vi "Weather Parse Test.vi"() -> ()   [LabVIEW 2020, in "CDM-Config.lvlib"] (continued)
        },\n                \"affectedZones\": [\n                    \"https://api.weather.gov/zones/forecast/PKZ760\"\n                ],\n                \"references\": [],\n                \"sent\": \"2025-12-03T04:00:00-09:00\",\n                \"effective\": \"2025-12-03T04:00:00-09:00\",\n                \"onset\": \"2025-12-03T04:00:00-09:00\",\n                \"expires\": \"2025-12-03T17:00:00-09:00\",\n                \"ends\": \"2025-12-04T17:00:00-09:00\",\n                \"status\": \"Actual\",\n                \"messageType\": \"Alert\",\n                \"category\": \"Met\",\n                \"severity\": \"Minor\",\n                \"certainty\": \"Likely\",\n                \"urgency\": \"Expected\",\n                \"event\": \"Small Craft Advisory\",\n                \"sender\": \"w-nws.webmaster@noaa.gov\",\n                \"senderName\": \"NWS Anchorage AK\",\n                \"headline\": \"Small Craft Advisory issued December 3 at 4:00AM AKST until December 4 at 5:00PM AKST by NWS Anchorage AK\",\n                \"description\": \"Coastal Waters Forecast for Southwest Alaska+Bristol Bay+The\\nAlaska Peninsula Waters and the Aleutian Islands up to 100 nm out.\\n\\nWind forecasts reflect the predominant speed and direction\\nexpected. Sea forecasts represent an average of the highest\\none-third of the combined wind wave and swell height.\\n\\n.TODAY...E wind 25 kt. Seas 5 ft.\\n.TONIGHT...E wind 30 kt. Seas 5 ft. Rain showers.\\n.THU...NE wind 30 kt. Seas 7 ft.\\n.THU NIGHT...NE wind 25 kt. Seas 7 ft.\\n.FRI...N wind 30 kt. Seas 6 ft.\\n.SAT...N wind 35 kt. Seas 9 ft.\\n.SUN...N wind 30 kt. Seas 7 ft.\",\n                \"instruction\": null,\n                \"response\": \"Avoid\",\n                \"parameters\": {\n                    \"AWIPSidentifier\": [\n                        \"CWFALU\"\n                    ],\n                    \"WMOidentifier\": [\n                        \"FZAK52 PAFC 031300\"\n                    ],\n                    \"NWSheadline\": [\n                        \"SMALL CRAFT ADVISORY THROUGH THURSDAY\"\n                    ],\n                    \"BLOCKCHANNEL\": [\n                        \"EAS\",\n                        \"NWEM\",\n                        \"CMAS\"\n                    ],\n                    \"VTEC\": [\n                        \"/O.NEW.PAFC.SC.Y.5665.251203T1300Z-251205T0200Z/\"\n                    ],\n                    \"eventEndingTime\": [\n                        \"2025-12-04T17:00:00-09:00\"\n                    ]\n                },\n                \"scope\": \"Public\",\n                \"code\": \"IPAWSv1.0\",\n                \"language\": \"en-US\",\n                \"web\": \"http://www.weather.gov\",\n                \"eventCode\": {\n                    \"SAME\": [\n                        \"NWS\"\n                    ],\n                    \"NationalWeatherService\": [\n                        \"SCY\"\n                    ]\n                }\n            }\n        },\n        {\n            \"id\": \"https://api.weather.gov/alerts/urn:oid:2.49.0.1.840.0.16ee1729296b80b5948b72c512c8722f6075ae6c.032.1\",\n            \"type\": \"Feature\",\n            \"geometry\": null,\n            \"properties\": {\n                \"@id\": \"https://api.weather.gov/alerts/urn:oid:2.49.0.1.840.0.16ee1729296b80b5948b72c512c8722f6075ae6c.032.1\",\n                \"@type\": \"wx:Alert\",\n                \"id\": \"urn:oid:2.49.0.1.840.0.16ee1729296b80b5948b72c512c8722f6075ae6c.032.1\",\n                \"areaDesc\": \"Bristol Bay from Cape Chichagof to Cape Pierce out to 15 NM\",\n                \"geocode\": {\n                    \"SAME\": [\n                        \"058762\"\n                    ],\n                    \"UGC\": [\n                        \"PKZ762\"\n                    ]\n                },\n                \"affectedZones\": [\n                    \"https://api.weather.gov/zones/forecast/PKZ762\"\n                ],\n                \"references\": [],\n                \"sent\": \"2025-12-03T04:00:00-09:00\",\n                \"effective\": \"2025-12-03T04:00:00-09:00\",\n                \"onset\": \"2025-12-03T17:00:00-09:00\",\n                \"expires\": \"2025-12-03T17:00:00-09:00\",\n                \"ends\": \"2025-12-04T17:00:00-09:00\",\n                \"status\": \"Actual\",\n                \"messageType\": \"Alert\",\n                \"category\": \"Met\",\n                \"severity\": \"Minor\",\n                \"certainty\": \"Likely\",\n                \"urgency\": \"Expected\",\n                \"event\": \"Small Craft Advisory\",\n                \"sender\": \"w-nws.webmaster@noaa.gov\",\n                \"senderName\": \"NWS Anchorage AK\",\n                \"headline\": \"Small Craft Advisory issued December 3 at 4:00AM AKST until December 4 at 5:00PM AKST by NWS Anchorage AK\",\n                \"description\": \"Coastal Waters Forecast for Southwest Alaska+Bristol Bay+The\\nAlaska Peninsula Waters and the Aleutian Islands up to 100 nm out.\\n\\nWind forecasts reflect the predominant speed and direction\\nexpected. Sea forecasts represent an average of the highest\\none-third of the combined wind wave and swell height.\\n\\n.TODAY...NE wind 20 kt. Seas 3 ft.\\n.TONIGHT...NE wind 25 kt. Seas 4 ft. Rain showers.\\n.THU...NE wind 25 kt. Seas 4 ft.\\n.THU NIGHT...NE wind 25 kt. Seas 4 ft.\\n.FRI...N wind 30 kt. Seas 4 ft.\\n.SAT...N wind 35 kt. Seas 5 ft.\\n.SUN...N wind 30 kt. Seas 3 ft.\",\n                \"instruction\": null,\n                \"response\": \"Avoid\",\n                \"parameters\": {\n                    \"AWIPSidentifier\": [\n                        \"CWFALU\"\n                    ],\n                    \"WMOidentifier\": [\n                        \"FZAK52 PAFC 031300\"\n                    ],\n                    \"NWSheadline\": [\n                        \"SMALL CRAFT ADVISORY TONIGHT AND THURSDAY\"\n                    ],\n                    \"BLOCKCHANNEL\": [\n                        \"EAS\",\n                        \"NWEM\",\n                        \"CMAS\"\n                    ],\n                    \"VTEC\": [\n                        \"/O.NEW.PAFC.SC.Y.5666.251204T0200Z-251205T0200Z/\"\n                    ],\n                    \"eventEndingTime\": [\n                        \"2025-12-04T17:00:00-09:00\"\n                    ]\n                },\n                \"scope\": \"Public\",\n                \"code\": \"IPAWSv1.0\",\n                \"language\": \"en-US\",\n                \"web\": \"http://www.weather.gov\",\n                \"eventCode\": {\n                    \"SAME\": [\n                        \"NWS\"\n                    ],\n                    \"NationalWeatherService\": [\n                        \"SCY\"\n                    ]\n                }\n            }\n        },\n        {\n            \"id\": \"https://api.weather.gov/alerts/urn:oid:2.49.0.1.840.0.16ee1729296b80b5948b72c512c8722f6075ae6c.011.1\",\n            \"type\": \"Feature\",\n            \"geometry\": null,\n            \"properties\": {\n                \"@id\": \"https://api.weather.gov/alerts/urn:oid:2.49.0.1.840.0.16ee1729296b80b5948b72c512c8722f6075ae6c.011.1\",\n                \"@type\": \"wx:Alert\",\n                \"id\": \"urn:oid:2.49.0.1.840.0.16ee1729296b80b5948b72c512c8722f6075ae6c.011.1\",\n                \"areaDesc\": \"Nelson Lagoon to Cape Sarichef from 15 to 70 NM\",\n                \"geocode\": {\n                    \"SAME\": [\n                        \"058759\"\n                    ],\n                    \"UGC\": [\n                        \"PKZ759\"\n                    ]\n                },\n                \"affectedZones\": [\n                    \"https://api.weather.gov/zones/forecast/PKZ759\"\n                ],\n                \"references\": [],\n                \"sent\": \"2025-12-03T04:00:00-09:00\",\n                \"effective\": \"2025-12-03T04:00:00-09:00\",\n                \"onset\": \"2025-12-03T04:00:00-09:00\",\n                \"expires\": \"2025-12-03T17:00:00-09:00\",\n                \"ends\": \"2025-12-04T17:00:00-09:00\",\n                \"status\": \"Actual\",\n                \"messageType\": \"Alert\",\n                \"category\": \"Met\",\n                \"severity\": \"Minor\",\n                \"certainty\": \"Likely\",\n                \"urgency\": \"Expected\",\n                \"event\": \"Small Craft Advisory\",\n                \"sender\": \"w-nws.webmaster@noaa.gov\",\n                \"senderName\": \"NWS Anchorage AK\",\n                \"headline\": \"Small Craft Advisory issued December 3 at 4:00AM AKST until December 4 at 5:00PM AKST by NWS Anchorage AK\",\n                \"description\": \"Coastal Waters Forecast for Southwest Alaska+Bristol Bay+The\\nAlaska Peninsula Waters and the Aleutian Islands up to 100 nm out.\\n\\nWind forecasts reflect the predominant speed and direction\\nexpected. Sea forecasts represent an average of the highest\\none-third of the combined wind wave and swell height.\\n\\n.TODAY...E wind 25 kt. Seas 9 ft. Rain showers.\\n.TONIGHT...NE wind 30 kt. Seas 11 ft. Rain showers.\\n.THU...NE wind 25 kt. Seas 12 ft.\\n.THU NIGHT...NE wind 25 kt. Seas 9 ft.\\n.FRI...NE wind 35 kt. Seas 12 ft.\\n.SAT...N wind 40 kt. Seas 17 ft.\\n.SUN...N wind 35 kt. Seas 16 ft.\",\n                \"instruction\": null,\n                \"response\": \"Avoid\",\n                \"parameters\": {\n                    \"AWIPSidentifier\": [\n                        \"CWFALU\"\n                    ],\n                    \"WMOidentifier\": [\n                        \"FZAK52 PAFC 031300\"\n                    ],\n                    \"NWSheadline\": [\n                        \"SMALL CRAFT ADVISORY THROUGH THURSDAY\"\n                    ],\n                    \"BLOCKCHANNEL\": [\n                        \"EAS\",\n                        \"NWEM\",\n                        \"CMAS\"\n                    ],\n                    \"VTEC\": [\n                        \"/O.NEW.PAFC.SC.Y.5646.251203T1300Z-251205T0200Z/\"\n                    ],\n                    \"eventEndingTime\": [\n                        \"2025-12-04T17:00:00-09:00\"\n                    ]\n                },\n                \"scope\": \"Public\",\n                \"code\": \"IPAWSv1.0\",\n                \"language\": \"en-US\",\n                \"web\": \"http://www.weather.gov\",\n                \"eventCode\": {\n                    \"SAME\": [\n                        \"NWS\"\n                    ],\n                    \"NationalWeatherService\": [\n                        \"SCY\"\n                    ]\n                }\n            }\n        },\n        {\n            \"id\": \"https://api.weather.gov/alerts/urn:oid:2.49.0.1.840.0.16ee1729296b80b5948b72c512c8722f6075ae6c.016.1\",\n            \"type\": \"Feature\",\n            \"geometry\": null,\n            \"properties\": {\n                \"@id\": \"https://api.weather.gov/alerts/urn:oid:2.49.0.1.840.0.16ee1729296b80b5948b72c512c8722f6075ae6c.016.1\",\n                \"@type\": \"wx:Alert\",\n                \"id\": \"urn:oid:2.49.0.1.840.0.16ee1729296b80b5948b72c512c8722f6075ae6c.016.1\",\n                \"areaDesc\": \"Cape Sarichef to Nikoski Pacific Side from 15 to 85 NM\",\n                \"geocode\": {\n                    \"SAME\": [\n                        \"058774\"\n                    ],\n                    \"UGC\": [\n                        \"PKZ774\"\n                    ]\n                },\n                \"affectedZones\": [\n                    \"https://api.weather.gov/zones/forecast/PKZ774\"\n                ],\n                \"references\": [],\n                \"sent\": \"2025-12-03T04:00:00-09:00\",\n                \"effective\": \"2025-12-03T04:00:00-09:00\",\n                \"onset\": \"2025-12-03T04:00:00-09:00\",\n                \"expires\": \"2025-12-03T17:00:00-09:00\",\n                \"ends\": \"2025-12-04T17:00:00-09:00\",\n                \"status\": \"Actual\",\n                \"messageType\": \"Alert\",\n                \"category\": \"Met\",\n                \"severity\": \"Minor\",\n                \"certainty\": \"Likely\",\n                \"urgency\": \"Expected\",\n                \"event\": \"Small Craft Advisory\",\n                \"sender\": \"w-nws.webmaster@noaa.gov\",\n                \"senderName\": \"NWS Anchorage AK\",\n                \"headline\": \"Small Craft Advisory issued December 3 at 4:00AM AKST until December 4 at 5:00PM AKST by NWS Anchorage AK\",\n                \"description\": \"Coastal Waters Forecast for Southwest Alaska+Bristol Bay+The\\nAlaska Peninsula Waters and the Aleutian Islands up to 100 nm out.\\n\\nWind forecasts reflect the predominant speed and direction\\nexpected. Sea forecasts represent an average of the highest\\none-third of the combined wind wave and swell height.\\n\\n.TODAY...E wind 25 kt. Seas 16 ft.\\n.TONIGHT...N wind 25 kt. Seas 10 ft.\\n.THU...N wind 25 kt. Seas 9 ft.\\n.THU NIGHT...NE wind 15 kt. Seas 6 ft.\\n.FRI...SW wind 25 kt. Seas 6 ft.\\n.SAT...NW wind 35 kt. Seas 11 ft.\\n.SUN...N wind 30 kt. Seas 10 ft.\",\n                \"instruction\": null,\n                \"response\": \"Avoid\",\n                \"parameters\": {\n                    \"AWIPSidentifier\": [\n                        \"CWFALU\"\n                    ],\n                    \"WMOidentifier\": [\n                        \"FZAK52 PAFC 031300\"\n                    ],\n                    \"NWSheadline\": [\n                        \"SMALL CRAFT ADVISORY THROUGH THURSDAY\"\n                    ],\n                    \"BLOCKCHANNEL\": [\n                        \"EAS\",\n                        \"NWEM\",\n                        \"CMAS\"\n                    ],\n                    \"VTEC\": [\n                        \"/O.NEW.PAFC.SC.Y.5651.251203T1300Z-251205T0200Z/\"\n                    ],\n                    \"eventEndingTime\": [\n                        \"2025-12-04T17:00:00-09:00\"\n                    ]\n                },\n                \"scope\": \"Public\",\n                \"code\": \"IPAWSv1.0\",\n                \"language\": \"en-US\",\n                \"web\": \"http://www.weather.gov\",\n                \"eventCode\": {\n                    \"SAME\": [\n                        \"NWS\"\n                    ],\n                    \"NationalWeatherService\": [\n                        \"SCY\"\n                    ]\n                }\n            }\n        },\n        {\n            \"id\": \"https://api.weather.gov/alerts/urn:oid:2.49.0.1.840.0.16ee1729296b80b5948b72c512c8722f6075ae6c.017.1\",\n            \"type\": \"Feature\",\n            \"geometry\": null,\n            \"properties\": {\n                \"@id\": \"https://api.weather.gov/alerts/urn:oid:2.49.0.1.840.0.16ee1729296b80b5948b72c512c8722f6075ae6c.017.1\",\n                \"@type\": \"wx:Alert\",\n                \"id\": \"urn:oid:2.49.0.1.840.0.16ee1729296b80b5948b72c512c8722f6075ae6c.017.1\",\n                \"areaDesc\": \"Nikolski to Seguam Bering Side out to 15 NM\",\n                \"geocode\": {\n                    \"SAME\": [\n                        \"058775\"\n                    ],\n                    \"UGC\": [\n                        \"PKZ775\"\n                    ]\n                },\n                \"affectedZones\": [\n                    \"https://api.weather.gov/zones/forecast/PKZ775\"\n                ],\n                \"references\": [],\n                \"sent\": \"2025-12-03T04:00:00-09:00\",\n                \"effective\": \"2025-12-03T04:00:00-09:00\",\n                \"onset\": \"2025-12-03T05:00:00-09:00\",\n                \"expires\": \"2025-12-03T17:00:00-09:00\",\n                \"ends\": \"2025-12-03T17:00:00-09:00\",\n                \"status\": \"Actual\",\n                \"messageType\": \"Alert\",\n                \"category\": \"Met\",\n                \"severity\": \"Moderate\",\n                \"certainty\": \"Likely\",\n                \"urgency\": \"Expected\",\n                \"event\": \"Gale Warning\",\n                \"sender\": \"w-nws.webmaster@noaa.gov\",\n                \"senderName\": \"NWS Anchorage AK\",\n                \"headline\": \"Gale Warning issued December 3 at 4:00AM AKST until December 3 at 5:00PM AKST by NWS Anchorage AK\",\n                \"description\": \"Coastal Waters Forecast for Southwest Alaska+Bristol Bay+The\\nAlaska Peninsula Waters and the Aleutian Islands up to 100 nm out.\\n\\nWind forecasts reflect the predominant speed and direction\\nexpected. Sea forecasts represent an average of the highest\\none-third of the combined wind wave and swell height.\\n\\n.TODAY...N wind 35 kt. Seas 23 ft. Rain.\\n.TONIGHT...N wind 30 kt. Seas 22 ft.\\n.THU...N wind 30 kt. Seas 16 ft.\\n.THU NIGHT...NE wind 20 kt. Seas 11 ft.\\n.FRI...E wind 20 kt. Seas 7 ft.\\n.SAT...N wind 30 kt. Seas 11 ft.\\n.SUN...N wind 30 kt. Seas 20 ft.\",\n                \"instruction\": null,\n                \"response\": \"Avoid\",\n                \"parameters\": {\n                    \"AWIPSidentifier\": [\n                        \"CWFALU\"\n                    ],\n                    \"WMOidentifier\": [\n                        \"FZAK52 PAFC 031300\"\n                    ],\n                    \"NWSheadline\": [\n                        \"GALE WARNING TODAY\"\n                    ],\n                    \"BLOCKCHANNEL\": [\n                        \"EAS\",\n                        \"NWEM\",\n                        \"CMAS\"\n                    ],\n                    \"VTEC\": [\n                        \"/O.NEW.PAFC.GL.W.5652.251203T1400Z-251204T0200Z/\"\n                    ],\n                    \"eventEndingTime\": [\n                        \"2025-12-03T17:00:00-09:00\"\n                    ]\n                },\n                \"scope\": \"Public\",\n                \"code\": \"IPAWSv1.0\",\n                \"language\": \"en-US\",\n                \"web\": \"http://www.weather.gov\",\n                \"eventCode\": {\n                    \"SAME\": [\n                        \"NWS\"\n                    ],\n                    \"NationalWeatherService\": [\n                        \"GLW\"\n                    ]\n                }\n            }\n        },\n        {\n            \"id\": \"https://api.weather.gov/alerts/urn:oid:2.49.0.1.840.0.16ee1729296b80b5948b72c512c8722f6075ae6c.014.1\",\n            \"type\": \"Feature\",\n            \"geometry\": null,\n            \"properties\": {\n                \"@id\": \"https://api.weather.gov/alerts/urn:oid:2.49.0.1.840.0.16ee1729296b80b5948b72c512c8722f6075ae6c.014.1\",\n                \"@type\": \"wx:Alert\",\n                \"id\": \"urn:oid:2.49.0.1.840.0.16ee1729296b80b5948b72c512c8722f6075ae6c.014.1\",\n                \"areaDesc\": \"Unalaska Bay\",\n                \"geocode\": {\n                    \"SAME\": [\n                        \"058771\"\n                    ],\n                    \"UGC\": [\n                        \"PKZ771\"\n                    ]\n                },\n                \"affectedZones\": [\n                    \"https://api.weather.gov/zones/forecast/PKZ771\"\n                ],\n                \"references\": [],\n                \"sent\": \"2025-12-03T04:00:00-09:00\",\n                \"effective\": \"2025-12-03T04:00:00-09:00\",\n                \"onset\": \"2025-12-03T05:00:00-09:00\",\n                \"expires\": \"2025-12-03T17:00:00-09:00\",\n                \"ends\": \"2025-12-03T17:00:00-09:00\",\n                \"status\": \"Actual\",\n                \"messageType\": \"Alert\",\n                \"category\": \"Met\",\n                \"severity\": \"Minor\",\n                \"certainty\": \"Likely\",\n                \"urgency\": \"Expected\",\n                \"event\": \"Small Craft Advisory\",\n                \"sender\": \"w-nws.webmaster@noaa.gov\",\n                \"senderName\": \"NWS Anchorage AK\",\n                \"headline\": \"Small Craft Advisory issued December 3 at 4:00AM AKST until December 3 at 5:00PM AKST by NWS Anchorage AK\",\n                \"description\": \"Coastal Waters Forecast for Southwest Alaska+Bristol Bay+The\\nAlaska Peninsula Waters and the Aleutian Islands up to 100 nm out.\\n\\nWind forecasts reflect the predominant speed and direction\\nexpected. Sea forecasts represent an average of the highest\\none-third of the combined wind wave and swell height.\\n\\n.TODAY...NE wind 25 kt becoming N 15 kt in the afternoon. Seas 7\\nft. Rain showers.\\n.TONIGHT...N wind 20 kt. Seas 7 ft. Rain showers.\\n.THU...N wind 20 kt. Seas 7 ft. Rain showers.\\n.THU NIGHT...NE wind 15 kt. Seas 5 ft.\\n.FRI...NE wind 20 kt. Seas 5 ft.\\n.SAT THROUGH SUN...N wind 25 kt. Seas 10 ft.\",\n                \"instruction\": null,\n                \"response\": \"Avoid\",\n                \"parameters\": {\n                    \"AWIPSidentifier\": [\n                        \"CWFALU\"\n                    ],\n                    \"WMOidentifier\": [\n                        \"FZAK52 PAFC 031300\"\n                    ],\n                    \"NWSheadline\": [\n                        \"SMALL CRAFT ADVISORY TODAY\"\n                    ],\n                    \"BLOCKCHANNEL\": [\n                        \"EAS\",\n                        \"NWEM\",\n                        \"CMAS\"\n                    ],\n                    \"VTEC\": [\n                        \"/O.NEW.PAFC.SC.Y.5649.251203T1400Z-251204T0200Z/\"\n                    ],\n                    \"eventEndingTime\": [\n                        \"2025-12-03T17:00:00-09:00\"\n                    ]\n                },\n                \"scope\": \"Public\",\n                \"code\": \"IPAWSv1.0\",\n                \"language\": \"en-US\",\n                \"web\": \"http://www.weather.gov\",\n                \"eventCode\": {\n                    \"SAME\": [\n                        \"NWS\"\n                    ],\n                    \"NationalWeatherService\": [\n                        \"SCY\"\n                    ]\n                }\n            }\n        },\n        {\n            \"id\": \"https://api.weather.gov/alerts/urn:oid:2.49.0.1.840.0.16ee1729296b80b5948b72c512c8722f6075ae6c.035.1\",\n            \"type\": \"Feature\",\n            \"geometry\": null,\n            \"properties\": {\n                \"@id\": \"https://api.weather.gov/alerts/urn:oid:2.49.0.1.840.0.16ee1729296b80b5948b72c512c8722f6075ae6c.035.1\",\n                \"@type\": \"wx:Alert\",\n                \"id\": \"urn:oid:2.49.0.1.840.0.16ee1729296b80b5948b72c512c8722f6075ae6c.035.1\",\n                \"areaDesc\": \"North and West of Nunivak Island\",\n                \"geocode\": {\n                    \"SAME\": [\n                        \"058765\"\n                    ],\n                    \"UGC\": [\n                        \"PKZ765\"\n                    ]\n                },\n                \"affectedZones\": [\n                    \"https://api.weather.gov/zones/forecast/PKZ765\"\n                ],\n                \"references\": [],\n                \"sent\": \"2025-12-03T04:00:00-09:00\",\n                \"effective\": \"2025-12-03T04:00:00-09:00\",\n                \"onset\": \"2025-12-03T04:00:00-09:00\",\n                \"expires\": \"2025-12-03T17:00:00-09:00\",\n                \"ends\": \"2025-12-04T05:00:00-09:00\",\n                \"status\": \"Actual\",\n                \"messageType\": \"Alert\",\n                \"category\": \"Met\",\n                \"severity\": \"Moderate\",\n                \"certainty\": \"Likely\",\n                \"urgency\": \"Expected\",\n                \"event\": \"Gale Warning\",\n                \"sender\": \"w-nws.webmaster@noaa.gov\",\n                \"senderName\": \"NWS Anchorage AK\",\n                \"headline\": \"Gale Warning issued December 3 at 4:00AM AKST until December 4 at 5:00AM AKST by NWS Anchorage AK\",\n                \"description\": \"Coastal Waters Forecast for Southwest Alaska+Bristol Bay+The\\nAlaska Peninsula Waters and the Aleutian Islands up to 100 nm out.\\n\\nWind forecasts reflect the predominant speed and direction\\nexpected. Sea forecasts represent an average of the highest\\none-third of the combined wind wave and swell height.\\n\\n.TODAY...NE wind 40 kt. Seas 14 ft. Freezing spray.\\n.TONIGHT...N wind 35 kt. Seas 11 ft. Freezing spray.\\n.THU...NE wind 30 kt. Seas 8 ft. Freezing spray.\\n.THU NIGHT...NE wind 25 kt. Seas 6 ft.\\n.FRI...NE wind 25 kt. Seas 6 ft.\\n.SAT...N wind 35 kt. Seas 14 ft.\\n.SUN...N wind 40 kt. Seas 15 ft.\",\n                \"instruction\": null,\n                \"response\": \"Avoid\",\n                \"parameters\": {\n                    \"AWIPSidentifier\": [\n                        \"CWFALU\"\n                    ],\n                    \"WMOidentifier\": [\n                        \"FZAK52 PAFC 031300\"\n                    ],\n                    \"NWSheadline\": [\n                        \"GALE WARNING THROUGH TONIGHT\"\n                    ],\n                    \"BLOCKCHANNEL\": [\n                        \"EAS\",\n                        \"NWEM\",\n                        \"CMAS\"\n                    ],\n                    \"VTEC\": [\n                        \"/O.NEW.PAFC.GL.W.5670.251203T1300Z-251204T1400Z/\"\n                    ],\n                    \"eventEndingTime\": [\n                        \"2025-12-04T05:00:00-09:00\"\n                    ]\n                },\n                \"scope\": \"Public\",\n                \"code\": \"IPAWSv1.0\",\n                \"language\": \"en-US\",\n                \"web\": \"http://www.weather.gov\",\n                \"eventCode\": {\n                    \"SAME\": [\n                        \"NWS\"\n                    ],\n                    \"NationalWeatherService\": [\n                        \"GLW\"\n                    ]\n                }\n            }\n        },\n        {\n            \"id\": \"https://api.weather.gov/alerts/urn:oid:2.49.0.1.840.0.16ee1729296b80b5948b72c512c8722f6075ae6c.033.1\",\n            \"type\": \"Feature\",\n            \"geometry\": null,\n            \"properties\": {\n                \"@id\": \"https://api.weather.gov/alerts/urn:oid:2.49.0.1.840.0.16ee1729296b80b5948b72c512c8722f6075ae6c.033.1\",\n                \"@type\": \"wx:Alert\",\n                \"id\": \"urn:oid:2.49.0.1.840.0.16ee1729296b80b5948b72c512c8722f6075ae6c.033.1\",\n                \"areaDesc\": \"Kuskokwim Delta and Etolin Strait out to 15 NM\",\n                \"geocode\": {\n                    \"SAME\": [\n                        \"058763\"\n                    ],\n                    \"UGC\": [\n                        \"PKZ763\"\n                    ]\n                },\n                \"affectedZones\": [\n                    \"https://api.weather.gov/zones/forecast/PKZ763\"\n                ],\n                \"references\": [],\n                \"sent\": \"2025-12-03T04:00:00-09:00\",\n                \"effective\": \"2025-12-03T04:00:00-09:00\",\n                \"onset\": \"2025-12-03T04:00:00-09:00\",\n                \"expires\": \"2025-12-03T17:00:00-09:00\",\n                \"ends\": \"2025-12-04T17:00:00-09:00\",\n                \"status\": \"Actual\",\n                \"messageType\": \"Alert\",\n                \"category\": \"Met\",\n                \"severity\": \"Severe\",\n                \"certainty\": \"Likely\",\n                \"urgency\": \"Expected\",\n                \"event\": \"Heavy Freezing Spray Warning\",\n                \"sender\": \"w-nws.webmaster@noaa.gov\",\n                \"senderName\": \"NWS Anchorage AK\",\n                \"headline\": \"Heavy Freezing Spray Warning issued December 3 at 4:00AM AKST until December 4 at 5:00PM AKST by NWS Anchorage AK\",\n                \"description\": \"Coastal Waters Forecast for Southwest Alaska+Bristol Bay+The\\nAlaska Peninsula Waters and the Aleutian Islands up to 100 nm out.\\n\\nWind forecasts reflect the predominant speed and direction\\nexpected. Sea forecasts represent an average of the highest\\none-third of the combined wind wave and swell height.\\n\\n.TODAY...NE wind 25 kt. Seas in ice free waters 4 ft. Heavy freezing\\nspray.\\n.TONIGHT...N wind 30 kt. Seas in ice free waters 4 ft. Heavy\\nfreezing spray.\\n.THU...N wind 25 kt. Seas in ice free waters 4 ft. Heavy freezing\\nspray.\\n.THU NIGHT...NE wind 25 kt. Seas in ice free waters 3 ft.\\n.FRI...N wind 40 kt. Seas in ice free waters 5 ft.\\n.SAT...N wind 45 kt. Seas in ice free waters 7 ft.\\n.SUN...N wind 40 kt. Seas in ice free waters 6 ft.\",\n                \"instruction\": null,\n                \"response\": \"Avoid\",\n                \"parameters\": {\n                    \"AWIPSidentifier\": [\n                        \"CWFALU\"\n                    ],\n                    \"WMOidentifier\": [\n                        \"FZAK52 PAFC 031300\"\n                    ],\n                    \"NWSheadline\": [\n                        \"HEAVY FREEZING SPRAY WARNING THROUGH THURSDAY... ...SMALL CRAFT ADVISORY THROUGH THURSDAY\"\n                    ],\n                    \"BLOCKCHANNEL\": [\n                        \"EAS\",\n                        \"NWEM\",\n                        \"CMAS\"\n                    ],\n                    \"VTEC\": [\n                        \"/O.NEW.PAFC.UP.W.5667.251203T1300Z-251205T0200Z/\"\n                    ],\n                    \"eventEndingTime\": [\n                        \"2025-12-04T17:00:00-09:00\"\n                    ]\n                },\n                \"scope\": \"Public\",\n                \"code\": \"IPAWSv1.0\",\n                \"language\": \"en-US\",\n                \"web\": \"http://www.weather.gov\",\n                \"eventCode\": {\n                    \"SAME\": [\n                        \"NWS\"\n                    ],\n                    \"NationalWeatherService\": [\n                        \"UPW\"\n                    ]\n                }\n            }\n        },\n        {\n            \"id\": \"https://api.weather.gov/alerts/urn:oid:2.49.0.1.840.0.6ff70be9ff46d8360260666474121956b1c90d94.003.1\",\n            \"type\": \"Feature\",\n            \"geometry\": null,\n            \"properties\": {\n                \"@id\": \"https://api.weather.gov/alerts/urn:oid:2.49.0.1.840.0.6ff70be9ff46d8360260666474121956b1c90d94.003.1\",\n                \"@type\": \"wx:Alert\",\n                \"id\": \"urn:oid:2.49.0.1.840.0.6ff70be9ff46d8360260666474121956b1c90d94.003.1\",\n                \"areaDesc\": \"Bering Sea Offshore 171W to 180 and North of 56N\",\n                \"geocode\": {\n                    \"SAME\": [\n                        \"058412\"\n                    ],\n                    \"UGC\": [\n                        \"PKZ412\"\n                    ]\n                },\n                \"affectedZones\": [\n                    \"https://api.weather.gov/zones/forecast/PKZ412\"\n                ],\n                \"references\": [],\n                \"sent\": \"2025-12-03T04:00:00-09:00\",\n                \"effective\": \"2025-12-03T04:00:00-09:00\",\n                \"onset\": \"2025-12-03T04:00:00-09:00\",\n                \"expires\": \"2025-12-03T18:00:00-09:00\",\n                \"ends\": \"2025-12-04T05:00:00-09:00\",\n                \"status\": \"Actual\",\n                \"messageType\": \"Alert\",\n                \"category\": \"Met\",\n                \"severity\": \"Moderate\",\n                \"certainty\": \"Likely\",\n                \"urgency\": \"Expected\",\n                \"event\": \"Gale Warning\",\n                \"sender\": \"w-nws.webmaster@noaa.gov\",\n                \"senderName\": \"NWS Anchorage AK\",\n                \"headline\": \"Gale Warning issued December 3 at 4:00AM AKST until December 4 at 5:00AM AKST by NWS Anchorage AK\",\n                \"description\": \"Offshore Waters Forecast for the Bering Sea\\n\\nWind forecasts reflect the predominant speed and direction\\nexpected. Sea forecasts represent an average of the highest\\none-third of the combined wind wave and swell height.\\n\\n.TODAY...N wind 30 to 45 kt. Seas 16 to 24 ft.\\n.TONIGHT...NE wind 25 to 40 kt. Seas 10 to 18 ft.\\n.THU...NE wind 20 to 30 kt. Seas 8 to 13 ft.\\n.THU NIGHT...E wind 25 kt. Seas 7 to 10 ft.\\n.FRI THROUGH SAT...NE wind 10 to 25 kt. Seas 7 to 11 ft.\\n.SUN...NE wind 20 to 35 kt. Seas 11 to 19 ft.\",\n                \"instruction\": null,\n                \"response\": \"Avoid\",\n                \"parameters\": {\n                    \"AWIPSidentifier\": [\n                        \"OFFALU\"\n                    ],\n                    \"WMOidentifier\": [\n                        \"FZAK62 PAFC 031300\"\n                    ],\n                    \"NWSheadline\": [\n                        \"GALE WARNING THROUGH TONIGHT\"\n                    ],\n                    \"BLOCKCHANNEL\": [\n                        \"EAS\",\n                        \"NWEM\",\n                        \"CMAS\"\n                    ],\n                    \"VTEC\": [\n                        \"/O.NEW.PAFC.GL.W.9377.251203T1300Z-251204T1400Z/\"\n                    ],\n                    \"eventEndingTime\": [\n                        \"2025-12-04T05:00:00-09:00\"\n                    ]\n                },\n                \"scope\": \"Public\",\n                \"code\": \"IPAWSv1.0\",\n                \"language\": \"en-US\",\n                \"web\": \"http://www.weather.gov\",\n                \"eventCode\": {\n                    \"SAME\": [\n                        \"NWS\"\n                    ],\n                    \"NationalWeatherService\": [\n                        \"GLW\"\n                    ]\n                }\n            }\n        },\n        {\n            \"id\": \"https://api.weather.gov/alerts/urn:oid:2.49.0.1.840.0.6ff70be9ff46d8360260666474121956b1c90d94.005.1\",\n            \"type\": \"Feature\",\n            \"geometry\": null,\n            \"properties\": {\n                \"@id\": \"https://api.weather.gov/alerts/urn:oid:2.49.0.1.840.0.6ff70be9ff46d8360260666474121956b1c90d94.005.1\",\n                \"@type\": \"wx:Alert\",\n                \"id\": \"urn:oid:2.49.0.1.840.0.6ff70be9ff46d8360260666474121956b1c90d94.005.1\",\n                \"areaDesc\": \"Bering Sea Offshore East of 171W\",\n                \"geocode\": {\n                    \"SAME\": [\n                        \"058414\"\n                    ],\n                    \"UGC\": [\n                        \"PKZ414\"\n                    ]\n                },\n                \"affectedZones\": [\n                    \"https://api.weather.gov/zones/forecast/PKZ414\"\n                ],\n                \"references\": [],\n                \"sent\": \"2025-12-03T04:00:00-09:00\",\n                \"effective\": \"2025-12-03T04:00:00-09:00\",\n                \"onset\": \"2025-12-03T04:00:00-09:00\",\n                \"expires\": \"2025-12-03T18:00:00-09:00\",\n                \"ends\": \"2025-12-04T05:00:00-09:00\",\n                \"status\": \"Actual\",\n                \"messageType\": \"Alert\",\n                \"category\": \"Met\",\n                \"severity\": \"Moderate\",\n                \"certainty\": \"Likely\",\n                \"urgency\": \"Expected\",\n                \"event\": \"Gale Warning\",\n                \"sender\": \"w-nws.webmaster@noaa.gov\",\n                \"senderName\": \"NWS Anchorage AK\",\n                \"headline\": \"Gale Warning issued December 3 at 4:00AM AKST until December 4 at 5:00AM AKST by NWS Anchorage AK\",\n                \"description\": \"Offshore Waters Forecast for the Bering Sea\\n\\nWind forecasts reflect the predominant speed and direction\\nexpected. Sea forecasts represent an average of the highest\\none-third of the combined wind wave and swell height.\\n\\n.TODAY...NE wind 25 to 40 kt. Seas 10 to 18 ft. Rain showers.\\n.TONIGHT...N wind 35 kt. Seas 10 to 17 ft.\\n.THU...NE wind 30 kt. Seas 9 to 14 ft.\\n.THU NIGHT...NE wind 25 kt. Seas 7 to 11 ft.\\n.FRI...NE wind 15 to 30 kt. Seas 6 to 11 ft.\\n.SAT...N wind 25 to 40 kt. Seas 9 to 14 ft.\\n.SUN...N wind 30 to 40 kt. Seas 14 to 21 ft.\",\n                \"instruction\": null,\n                \"response\": \"Avoid\",\n                \"parameters\": {\n                    \"AWIPSidentifier\": [\n                        \"OFFALU\"\n                    ],\n                    \"WMOidentifier\": [\n                        \"FZAK62 PAFC 031300\"\n                    ],\n                    \"NWSheadline\": [\n                        \"GALE WARNING THROUGH TONIGHT\"\n                    ],\n                    \"BLOCKCHANNEL\": [\n                        \"EAS\",\n                        \"NWEM\",\n                        \"CMAS\"\n                    ],\n                    \"VTEC\": [\n                        \"/O.NEW.PAFC.GL.W.9379.251203T1300Z-251204T1400Z/\"\n                    ],\n                    \"eventEndingTime\": [\n                        \"2025-12-04T05:00:00-09:00\"\n                    ]\n                },\n                \"scope\": \"Public\",\n                \"code\": \"IPAWSv1.0\",\n                \"language\": \"en-US\",\n                \"web\": \"http://www.weather.gov\",\n                \"eventCode\": {\n                    \"SAME\": [\n                        \"NWS\"\n                    ],\n                    \"NationalWeatherService\": [\n                        \"GLW\"\n                    ]\n                }\n            }\n        },\n        {\n            \"id\": \"https://api.weather.gov/alerts/urn:oid:2.49.0.1.840.0.6ff70be9ff46d8360260666474121956b1c90d94.002.1\",\n            \"type\": \"Feature\",\n            \"geometry\": null,\n            \"properties\": {\n                \"@id\": \"https://api.weather.gov/alerts/urn:oid:2.49.0.1.840.0.6ff70be9ff46d8360260666474121956b1c90d94.002.1\",\n                \"@type\": \"wx:Alert\",\n                \"id\": \"urn:oid:2.49.0.1.840.0.6ff70be9ff46d8360260666474121956b1c90d94.002.1\",\n                \"areaDesc\": \"Bering Sea Offshore  West of 180 and East of the International Date Line\",\n                \"geocode\": {\n                    \"SAME\": [\n                        \"058411\"\n                    ],\n                    \"UGC\": [\n                        \"PKZ411\"\n                    ]\n                },\n                \"affectedZones\": [\n                    \"https://api.weather.gov/zones/forecast/PKZ411\"\n                ],\n                \"references\": [],\n                \"sent\": \"2025-12-03T04:00:00-09:00\",\n                \"effective\": \"2025-12-03T04:00:00-09:00\",\n                \"onset\": \"2025-12-04T05:00:00-09:00\",\n                \"expires\": \"2025-12-03T18:00:00-09:00\",\n                \"ends\": \"2025-12-04T17:00:00-09:00\",\n                \"status\": \"Actual\",\n                \"messageType\": \"Alert\",\n                \"category\": \"Met\",\n                \"severity\": \"Moderate\",\n                \"certainty\": \"Likely\",\n                \"urgency\": \"Expected\",\n                \"event\": \"Gale Warning\",\n                \"sender\": \"w-nws.webmaster@noaa.gov\",\n                \"senderName\": \"NWS Anchorage AK\",\n                \"headline\": \"Gale Warning issued December 3 at 4:00AM AKST until December 4 at 5:00PM AKST by NWS Anchorage AK\",\n                \"description\": \"Offshore Waters Forecast for the Bering Sea\\n\\nWind forecasts reflect the predominant speed and direction\\nexpected. Sea forecasts represent an average of the highest\\none-third of the combined wind wave and swell height.\\n\\n.TODAY...NE wind 15 to 30 kt. Seas 13 to 21 ft.\\n.TONIGHT...E wind 15 to 30 kt. Seas 9 to 16 ft.\\n.THU...SE wind 25 to 40 kt. Seas 9 to 14 ft.\\n.THU NIGHT...SE wind 25 to 40 kt. Seas 9 to 17 ft.\\n.FRI...E wind 10 to 25 kt. Seas 9 to 15 ft.\\n.SAT...NE wind up to 20 kt. Seas 7 to 10 ft.\\n.SUN...NE wind 25 kt. Seas 7 to 12 ft.\",\n                \"instruction\": null,\n                \"response\": \"Avoid\",\n                \"parameters\": {\n                    \"AWIPSidentifier\": [\n                        \"OFFALU\"\n                    ],\n                    \"WMOidentifier\": [\n                        \"FZAK62 PAFC 031300\"\n                    ],\n                    \"NWSheadline\": [\n                        \"GALE WARNING THURSDAY\"\n                    ],\n                    \"BLOCKCHANNEL\": [\n                        \"EAS\",\n                        \"NWEM\",\n                        \"CMAS\"\n                    ],\n                    \"VTEC\": [\n                        \"/O.NEW.PAFC.GL.W.9376.251204T1400Z-251205T0200Z/\"\n                    ],\n                    \"eventEndingTime\": [\n                        \"2025-12-04T17:00:00-09:00\"\n                    ]\n                },\n                \"scope\": \"Public\",\n                \"code\": \"IPAWSv1.0\",\n                \"language\": \"en-US\",\n                \"web\": \"http://www.weather.gov\",\n                \"eventCode\": {\n                    \"SAME\": [\n                        \"NWS\"\n                    ],\n                    \"NationalWeatherService\": [\n                        \"GLW\"\n                    ]\n                }\n            }\n        },\n        {\n            \"id\": \"https://api.weather.gov/alerts/urn:oid:2.49.0.1.840.0.6ff70be9ff46d8360260666474121956b1c90d94.004.1\",\n            \"type\": \"Feature\",\n            \"geometry\": null,\n            \"properties\": {\n                \"@id\": \"https://api.weather.gov/alerts/urn:oid:2.49.0.1.840.0.6ff70be9ff46d8360260666474121956b1c90d94.004.1\",\n                \"@type\": \"wx:Alert\",\n                \"id\": \"urn:oid:2.49.0.1.840.0.6ff70be9ff46d8360260666474121956b1c90d94.004.1\",\n                \"areaDesc\": \"Bering Sea Offshore 171W to 180 and South of 56N\",\n                \"geocode\": {\n                    \"SAME\": [\n                        \"058413\"\n                    ],\n                    \"UGC\": [\n                        \"PKZ413\"\n                    ]\n                },\n                \"affectedZones\": [\n                    \"https://api.weather.gov/zones/forecast/PKZ413\"\n                ],\n                \"references\": [],\n                \"sent\": \"2025-12-03T04:00:00-09:00\",\n                \"effective\": \"2025-12-03T04:00:00-09:00\",\n                \"onset\": \"2025-12-03T04:00:00-09:00\",\n                \"expires\": \"2025-12-03T18:00:00-09:00\",\n                \"ends\": \"2025-12-04T05:00:00-09:00\",\n                \"status\": \"Actual\",\n                \"messageType\": \"Alert\",\n                \"category\": \"Met\",\n                \"severity\": \"Moderate\",\n                \"certainty\": \"Likely\",\n                \"urgency\": \"Expected\",\n                \"event\": \"Gale Warning\",\n                \"sender\": \"w-nws.webmaster@noaa.gov\",\n                \"senderName\": \"NWS Anchorage AK\",\n                \"headline\": \"Gale Warning issued December 3 at 4:00AM AKST until December 4 at 5:00AM AKST by NWS Anchorage AK\",\n                \"description\": \"Offshore Waters Forecast for the Bering Sea\\n\\nWind forecasts reflect the predominant speed and direction\\nexpected. Sea forecasts represent an average of the highest\\none-third of the combined wind wave and swell height.\\n\\n.TODAY...N wind 30 to 45 kt. Seas 20 to 28 ft.\\n.TONIGHT...N wind 20 to 35 kt. Seas 14 to 22 ft.\\n.THU...NE wind 15 to 30 kt. Seas 10 to 15 ft.\\n.THU NIGHT...E wind 15 to 25 kt. Seas 8 to 11 ft.\\n.FRI THROUGH SAT...NE wind 10 to 25 kt. Seas 6 to 10 ft.\\n.SUN...NE wind 30 kt. Seas 13 to 21 ft.\",\n                \"instruction\": null,\n                \"response\": \"Avoid\",\n                \"parameters\": {\n                    \"AWIPSidentifier\": [\n                        \"OFFALU\"\n                    ],\n                    \"WMOidentifier\": [\n                        \"FZAK62 PAFC 031300\"\n                    ],\n                    \"NWSheadline\": [\n                        \"GALE WARNING THROUGH TONIGHT\"\n                    ],\n                    \"BLOCKCHANNEL\": [\n                        \"EAS\",\n                        \"NWEM\",\n                        \"CMAS\"\n                    ],\n                    \"VTEC\": [\n                        \"/O.NEW.PAFC.GL.W.9378.251203T1300Z-251204T1400Z/\"\n                    ],\n                    \"eventEndingTime\": [\n                        \"2025-12-04T05:00:00-09:00\"\n                    ]\n                },\n                \"scope\": \"Public\",\n                \"code\": \"IPAWSv1.0\",\n                \"language\": \"en-US\",\n                \"web\": \"http://www.weather.gov\",\n                \"eventCode\": {\n                    \"SAME\": [\n                        \"NWS\"\n                    ],\n                    \"NationalWeatherService\": [\n                        \"GLW\"\n                    ]\n                }\n            }\n        },\n        {\n            \"id\": \"https://api.weather.gov/alerts/urn:oid:2.49.0.1.840.0.1c5cf705b4d7c500670d34f464b8d97f479637e0.016.1\",\n            \"type\": \"Feature\",\n            \"geometry\": null,\n            \"properties\": {\n                \"@id\": \"https://api.weather.gov/alerts/urn:oid:2.49.0.1.840.0.1c5cf705b4d7c500670d34f464b8d97f479637e0.016.1\",\n                \"@type\": \"wx:Alert\",\n                \"id\": \"urn:oid:2.49.0.1.840.0.1c5cf705b4d7c500670d34f464b8d97f479637e0.016.1\",\n                \"areaDesc\": \"Kwemeluk Pass to Kwikpak Pass from 15 to 90 NM\",\n                \"geocode\": {\n                    \"SAME\": [\n                        \"058853\"\n                    ],\n                    \"UGC\": [\n                        \"PKZ853\"\n                    ]\n                },\n                \"affectedZones\": [\n                    \"https://api.weather.gov/zones/forecast/PKZ853\"\n                ],\n                \"references\": [],\n                \"sent\": \"2025-12-03T03:47:00-09:00\",\n                \"effective\": \"2025-12-03T03:46:00-09:00\",\n                \"onset\": \"2025-12-03T03:00:00-09:00\",\n                \"expires\": \"2025-12-03T18:00:00-09:00\",\n                \"ends\": \"2025-12-04T05:00:00-09:00\",\n                \"status\": \"Actual\",\n                \"messageType\": \"Alert\",\n                \"category\": \"Met\",\n                \"severity\": \"Severe\",\n                \"certainty\": \"Likely\",\n                \"urgency\": \"Expected\",\n                \"event\": \"Heavy Freezing Spray Warning\",\n                \"sender\": \"w-nws.webmaster@noaa.gov\",\n                \"senderName\": \"NWS Fairbanks AK\",\n                \"headline\": \"Heavy Freezing Spray Warning issued December 3 at 3:46AM AKST until December 4 at 5:00AM AKST by NWS Fairbanks AK\",\n                \"description\": \"Northwestern Alaska Coastal Waters out 100 NM\\n\\nWind forecasts reflect the predominant speed and direction\\nexpected. Sea forecasts represent the average of the highest one-\\nthird of the combined wind-wave and swell height.\\n\\n.TODAY...N winds 35 kt. Seas 9 ft. Heavy freezing spray.\\n.TONIGHT...NE winds 20 kt. Seas 5 ft. Heavy freezing spray.\\n.THU...NE winds 15 kt. Seas 3 ft.\\n.THU NIGHT...NE winds 15 kt. Seas 2 ft.\\n.FRI...NE winds 10 kt. Seas 2 ft.\\n.FRI NIGHT...NE winds 20 kt. Seas 3 ft. Freezing spray.\\n.SAT...NE winds 30 kt. Seas 6 ft.\\n.SUN...NE winds 40 kt. Seas 7 ft.\",\n                \"instruction\": null,\n                \"response\": \"Avoid\",\n                \"parameters\": {\n                    \"AWIPSidentifier\": [\n                        \"CWFWCZ\"\n                    ],\n                    \"WMOidentifier\": [\n                        \"FZAK52 PAFG 031247\"\n                    ],\n                    \"NWSheadline\": [\n                        \"GALE WARNING IN EFFECT THROUGH EARLY THIS MORNING... ...HEAVY FREEZING SPRAY WARNING IN EFFECT THROUGH LATE TONIGHT\"\n                    ],\n                    \"BLOCKCHANNEL\": [\n                        \"EAS\",\n                        \"NWEM\",\n                        \"CMAS\"\n                    ],\n                    \"VTEC\": [\n                        \"/O.NEW.PAFG.UP.W.8908.251203T1200Z-251204T1400Z/\"\n                    ],\n                    \"eventEndingTime\": [\n                        \"2025-12-04T05:00:00-09:00\"\n                    ]\n                },\n                \"scope\": \"Public\",\n                \"code\": \"IPAWSv1.0\",\n                \"language\": \"en-US\",\n                \"web\": \"http://www.weather.gov\",\n                \"eventCode\": {\n                    \"SAME\": [\n                        \"NWS\"\n                    ],\n                    \"NationalWeatherService\": [\n                        \"UPW\"\n                    ]\n                }\n            }\n        },\n        {\n            \"id\": \"https://api.weather.gov/alerts/urn:oid:2.49.0.1.840.0.1c5cf705b4d7c500670d34f464b8d97f479637e0.011.1\",\n            \"type\": \"Feature\",\n            \"geometry\": null,\n            \"properties\": {\n                \"@id\": \"https://api.weather.gov/alerts/urn:oid:2.49.0.1.840.0.1c5cf705b4d7c500670d34f464b8d97f479637e0.011.1\",\n                \"@type\": \"wx:Alert\",\n                \"id\": \"urn:oid:2.49.0.1.840.0.1c5cf705b4d7c500670d34f464b8d97f479637e0.011.1\",\n                \"areaDesc\": \"South Side of Saint Lawrence Island out to 15 NM\",\n                \"geocode\": {\n                    \"SAME\": [\n                        \"058816\"\n                    ],\n                    \"UGC\": [\n                        \"PKZ816\"\n                    ]\n                },\n                \"affectedZones\": [\n                    \"https://api.weather.gov/zones/forecast/PKZ816\"\n                ],\n                \"references\": [],\n                \"sent\": \"2025-12-03T03:47:00-09:00\",\n                \"effective\": \"2025-12-03T03:46:00-09:00\",\n                \"onset\": \"2025-12-03T03:00:00-09:00\",\n                \"expires\": \"2025-12-03T18:00:00-09:00\",\n                \"ends\": \"2025-12-04T05:00:00-09:00\",\n                \"status\": \"Actual\",\n                \"messageType\": \"Alert\",\n                \"category\": \"Met\",\n                \"severity\": \"Severe\",\n                \"certainty\": \"Likely\",\n                \"urgency\": \"Expected\",\n                \"event\": \"Heavy Freezing Spray Warning\",\n                \"sender\": \"w-nws.webmaster@noaa.gov\",\n                \"senderName\": \"NWS Fairbanks AK\",\n                \"headline\": \"Heavy Freezing Spray Warning issued December 3 at 3:46AM AKST until December 4 at 5:00AM AKST by NWS Fairbanks AK\",\n                \"description\": \"Northwestern Alaska Coastal Waters out 100 NM\\n\\nWind forecasts reflect the predominant speed and direction\\nexpected. Sea forecasts represent the average of the highest one-\\nthird of the combined wind-wave and swell height.\\n\\n.TODAY...N winds 35 kt. Seas 8 ft subsiding to 6 ft. Heavy\\nfreezing spray.\\n.TONIGHT...N winds 20 kt. Seas 4 ft. Heavy freezing spray.\\n.THU...N winds 15 kt. Seas 3 ft. Freezing spray.\\n.THU NIGHT...N winds 10 kt. Seas 2 ft.\\n.FRI...NE winds 10 kt. Seas 2 ft.\\n.FRI NIGHT...NE winds 20 kt. Seas 5 ft. Heavy freezing spray.\\n.SAT...NE winds 30 kt. Seas 6 ft.\\n.SUN...NE winds 30 kt. Seas 7 ft.\",\n                \"instruction\": null,\n                \"response\": \"Avoid\",\n                \"parameters\": {\n                    \"AWIPSidentifier\": [\n                        \"CWFWCZ\"\n                    ],\n                    \"WMOidentifier\": [\n                        \"FZAK52 PAFG 031247\"\n                    ],\n                    \"NWSheadline\": [\n                        \"GALE WARNING IN EFFECT THROUGH EARLY THIS MORNING... ...HEAVY FREEZING SPRAY WARNING IN EFFECT THROUGH LATE TONIGHT\"\n                    ],\n                    \"BLOCKCHANNEL\": [\n                        \"EAS\",\n                        \"NWEM\",\n                        \"CMAS\"\n                    ],\n                    \"VTEC\": [\n                        \"/O.NEW.PAFG.UP.W.8905.251203T1200Z-251204T1400Z/\"\n                    ],\n                    \"eventEndingTime\": [\n                        \"2025-12-04T05:00:00-09:00\"\n                    ]\n                },\n                \"scope\": \"Public\",\n                \"code\": \"IPAWSv1.0\",\n                \"language\": \"en-US\",\n                \"web\": \"http://www.weather.gov\",\n                \"eventCode\": {\n                    \"SAME\": [\n                        \"NWS\"\n                    ],\n                    \"NationalWeatherService\": [\n                        \"UPW\"\n                    ]\n                }\n            }\n        },\n        {\n            \"id\": \"https://api.weather.gov/alerts/urn:oid:2.49.0.1.840.0.1c5cf705b4d7c500670d34f464b8d97f479637e0.013.1\",\n            \"type\": \"Feature\",\n            \"geometry\": null,\n            \"properties\": {\n                \"@id\": \"https://api.weather.gov/alerts/urn:oid:2.49.0.1.840.0.1c5cf705b4d7c500670d34f464b8d97f479637e0.013.1\",\n                \"@type\": \"wx:Alert\",\n                \"id\": \"urn:oid:2.49.0.1.840.0.1c5cf705b4d7c500670d34f464b8d97f479637e0.013.1\",\n                \"areaDesc\": \"Etolin Strait to Kwemeluk Pass from 15 to 90 NM\",\n                \"geocode\": {\n                    \"SAME\": [\n                        \"058850\"\n                    ],\n                    \"UGC\": [\n                        \"PKZ850\"\n                    ]\n                },\n                \"affectedZones\": [\n                    \"https://api.weather.gov/zones/forecast/PKZ850\"\n                ],\n                \"references\": [],\n                \"sent\": \"2025-12-03T03:47:00-09:00\",\n                \"effective\": \"2025-12-03T03:46:00-09:00\",\n                \"onset\": \"2025-12-03T03:00:00-09:00\",\n                \"expires\": \"2025-12-03T18:00:00-09:00\",\n                \"ends\": \"2025-12-04T05:00:00-09:00\",\n                \"status\": \"Actual\",\n                \"messageType\": \"Alert\",\n                \"category\": \"Met\",\n                \"severity\": \"Severe\",\n                \"certainty\": \"Likely\",\n                \"urgency\": \"Expected\",\n                \"event\": \"Heavy Freezing Spray Warning\",\n                \"sender\": \"w-nws.webmaster@noaa.gov\",\n                \"senderName\": \"NWS Fairbanks AK\",\n                \"headline\": \"Heavy Freezing Spray Warning issued December 3 at 3:46AM AKST until December 4 at 5:00AM AKST by NWS Fairbanks AK\",\n                \"description\": \"Northwestern Alaska Coastal Waters out 100 NM\\n\\nWind forecasts reflect the predominant speed and direction\\nexpected. Sea forecasts represent the average of the highest one-\\nthird of the combined wind-wave and swell height.\\n\\n.TODAY...N winds 35 kt. Seas 10 ft. Heavy freezing spray.\\n.TONIGHT...NE winds 35 kt. Seas 7 ft. Heavy freezing spray.\\n.THU...NE winds 20 kt. Seas 4 ft. Heavy freezing spray.\\n.THU NIGHT...NE winds 20 kt. Seas 4 ft. Heavy freezing spray.\\n.FRI...NE winds 15 kt. Seas 3 ft. Heavy freezing spray.\\n.FRI NIGHT...NE winds 20 kt. Seas 4 ft. Heavy freezing spray.\\n.SAT...NE winds 35 kt. Seas 7 ft.\\n.SUN...NE winds 40 kt. Seas 8 ft.\",\n                \"instruction\": null,\n                \"response\": \"Avoid\",\n                \"parameters\": {\n                    \"AWIPSidentifier\": [\n                        \"CWFWCZ\"\n                    ],\n                    \"WMOidentifier\": [\n                        \"FZAK52 PAFG 031247\"\n                    ],\n                    \"NWSheadline\": [\n                        \"GALE WARNING IN EFFECT THROUGH THIS AFTERNOON... ...HEAVY FREEZING SPRAY WARNING IN EFFECT THROUGH LATE TONIGHT\"\n                    ],\n                    \"BLOCKCHANNEL\": [\n                        \"EAS\",\n                        \"NWEM\",\n                        \"CMAS\"\n                    ],\n                    \"VTEC\": [\n                        \"/O.NEW.PAFG.UP.W.8906.251203T1200Z-251204T1400Z/\"\n                    ],\n                    \"eventEndingTime\": [\n                        \"2025-12-04T05:00:00-09:00\"\n                    ]\n                },\n                \"scope\": \"Public\",\n                \"code\": \"IPAWSv1.0\",\n                \"language\": \"en-US\",\n                \"web\": \"http://www.weather.gov\",\n                \"eventCode\": {\n                    \"SAME\": [\n                        \"NWS\"\n                    ],\n                    \"NationalWeatherService\": [\n                        \"UPW\"\n                    ]\n                }\n            }\n        },\n        {\n            \"id\": \"https://api.weather.gov/alerts/urn:oid:2.49.0.1.840.0.1c5cf705b4d7c500670d34f464b8d97f479637e0.014.1\",\n            \"type\": \"Feature\",\n            \"geometry\": null,\n            \"properties\": {\n                \"@id\": \"https://api.weather.gov/alerts/urn:oid:2.49.0.1.840.0.1c5cf705b4d7c500670d34f464b8d97f479637e0.014.1\",\n                \"@type\": \"wx:Alert\",\n                \"id\": \"urn:oid:2.49.0.1.840.0.1c5cf705b4d7c500670d34f464b8d97f479637e0.014.1\",\n                \"areaDesc\": \"Southwest of Saint Lawrence Island from 15 to 100 NM\",\n                \"geocode\": {\n                    \"SAME\": [\n                        \"058851\"\n                    ],\n                    \"UGC\": [\n                        \"PKZ851\"\n                    ]\n                },\n                \"affectedZones\": [\n                    \"https://api.weather.gov/zones/forecast/PKZ851\"\n                ],\n                \"references\": [],\n                \"sent\": \"2025-12-03T03:47:00-09:00\",\n                \"effective\": \"2025-12-03T03:46:00-09:00\",\n                \"onset\": \"2025-12-03T03:00:00-09:00\",\n                \"expires\": \"2025-12-03T18:00:00-09:00\",\n                \"ends\": \"2025-12-04T05:00:00-09:00\",\n                \"status\": \"Actual\",\n                \"messageType\": \"Alert\",\n                \"category\": \"Met\",\n                \"severity\": \"Severe\",\n                \"certainty\": \"Likely\",\n                \"urgency\": \"Expected\",\n                \"event\": \"Heavy Freezing Spray Warning\",\n                \"sender\": \"w-nws.webmaster@noaa.gov\",\n                \"senderName\": \"NWS Fairbanks AK\",\n                \"headline\": \"Heavy Freezing Spray Warning issued December 3 at 3:46AM AKST until December 4 at 5:00AM AKST by NWS Fairbanks AK\",\n                \"description\": \"Northwestern Alaska Coastal Waters out 100 NM\\n\\nWind forecasts reflect the predominant speed and direction\\nexpected. Sea forecasts represent the average of the highest one-\\nthird of the combined wind-wave and swell height.\\n\\n.TODAY...N winds 35 kt. Seas 10 ft. Heavy freezing spray.\\n.TONIGHT...N winds 25 kt. Seas 6 ft. Heavy freezing spray.\\n.THU...NE winds 15 kt. Seas 3 ft. Freezing spray.\\n.THU NIGHT...E winds 15 kt. Seas 3 ft.\\n.FRI...NE winds 15 kt. Seas 5 ft. Freezing spray.\\n.FRI NIGHT...NE winds 20 kt. Seas 6 ft. Freezing spray.\\n.SAT...NE winds 25 kt. Seas 8 ft.\\n.SUN...NE winds 35 kt. Seas 7 ft.\",\n                \"instruction\": null,\n        
